vi "Read Single Analog Channel.vi"() -> ()   [LabVIEW 2020]
uses:
  <instrlib>/BDAQ-6104/BDAQ-6104.lvlib
panel:
  out "Channel Data":dbl
  in  "Channel":T1(ring)
  in  "VISA resource name":refnum<visa-resource-name>
  # "Volts"
  # "Connect to the DAQ Module and read the specified\nchannel data. The default measurment value is in volts."
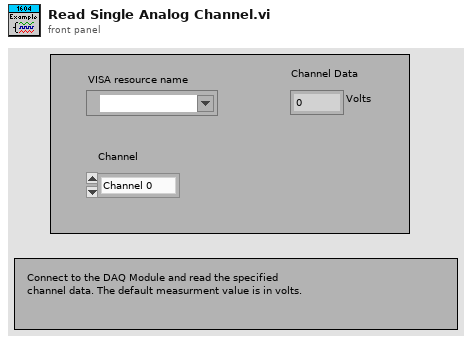
[diagram p1: front panel]
types:
  T1 = enum16{"Channel 0", "Channel 1", "Channel 2", "Channel 3", "Channel 4", "Channel 5"}
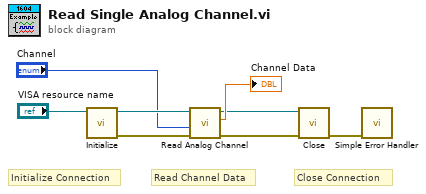
[diagram p0: block diagram]
diagram:
  # "Close Connection"
  # "Read Channel Data"
  # "Initialize Connection"
  n1 = call <instrlib>:"Initialize.vi"("VISA resource name"="VISA resource name") -> ("error out"=w7:errorcluster, "VISA resource name out"=w6:refnum<visa-resource-name>)  [unwired: 9 in]
  n2 = call-poly <instrlib>:"Read Analog Channel.vi"("error in (no error)"=w7, "Channel"="Channel", "VISA resource name"=w6) -> ("error out"=w3:errorcluster, "Channel Data"=→"Channel Data":dbl, "VISA resource name"=w2:refnum<visa-resource-name>)  [unwired: 6 in]
  n3 = call <instrlib>:"Close.vi"("error in (no error)"=w3, "VISA resource name"=w2) -> ("error out"=w1:errorcluster)  [unwired: 9 in]
  n4 = call <vilib>:"Simple Error Handler.vi"("error in (no error)"=w1) -> ()  [unwired: 4 in, 5 out]
